vi "Temp PID Control.vi"() -> ()   [LabVIEW 2018]
doc: "This example demonstrates how to generate digital output data using software timing.\n\nFor instructions on how to connect your signals from the DAQ device, refer to your device documentation."
uses:
  <vilib>/Utility/error.llb/DialogType.ctl
  <vilib>/DAQmx/write.llb/DAQmx Write (Digital Bool 1Line 1Point).vi
  <vilib>/DAQmx/create/channels.llb/DAQmx Create Channel (AI-Voltage-Basic).vi
  <vilib>/DAQmx/configure/timing.llb/DAQmx Timing (Sample Clock).vi
  <resource>/objmgr/daqmx.rc
  <vilib>/DAQmx/read.llb/DAQmx Read (Analog Wfm 1Chan NSamp).vi
  <vilib>/measure/NI_MAPro.lvlib
  <vilib>/measure/madcrms.llb/Basic Averaged DC-RMS for 1 Chan.vi
  <vilib>/addons/control/pid/NI_PID_pid.lvlib
  <vilib>/addons/control/pid/pid.llb/PID (DBL).vi
  <vilib>/DAQmx/create/channels.llb/DAQmx Create Channel (DO-Digital Output).vi
  <vilib>/DAQmx/write.llb/DAQmx Write (Digital 1D Bool NChan 1Samp 1Line).vi
panel:
  out "STOP":bool
  out "On Ratio [%]":dbl format="%.2f"
  in  "output range":cluster{"output high":dbl, "output low":dbl}={"output high"=100.0, "output low"=0.0} {"output low" format="%.2f"; "output high" format="%.2f"}
  in  "PID gains":T1={"proportional gain (Kc)"=1.0, "integral time (Ti, min)"=0.01, "derivative time (Td, min)"=0.0} {"derivative time (Td, min)" format="%.3f"; "integral time (Ti, min)" format="%.3f"; "proportional gain (Kc)" format="%.3f"}
  in  "Temperature Setpoint":dbl(slide) scale=20.0..100.0
  out "Average Temperature":dbl=1000.0 format="%0.2f"
  in  "Temperature Window Length in [s]":dbl=1000.0
  out "Waveform Graph":waveform(dbl)(graph)
  in  "Sample Rate":dbl=1000.0
  in  "Sample Clock Source":tag="OnboardClock"
  in  "Terminal Configuration":i32(ring)=-1 items=["default"=-1, "RSE"=10083, "NRSE"=10078, "Differential"=10106, "Pseudodifferential"=12529]
  in  "Max Voltage":dbl=5.0
  in  "Min Voltage":dbl=-5.0
  in  "Physical Channel":tag="Dev1/ai0"
  out "Actual Sample Rate":dbl=1000.0 format="%0.2f"
  in  "Stop":bool
  in  "Line(s)":tag="Dev1/port0/line0:1"
  # "Digital Output Channel"
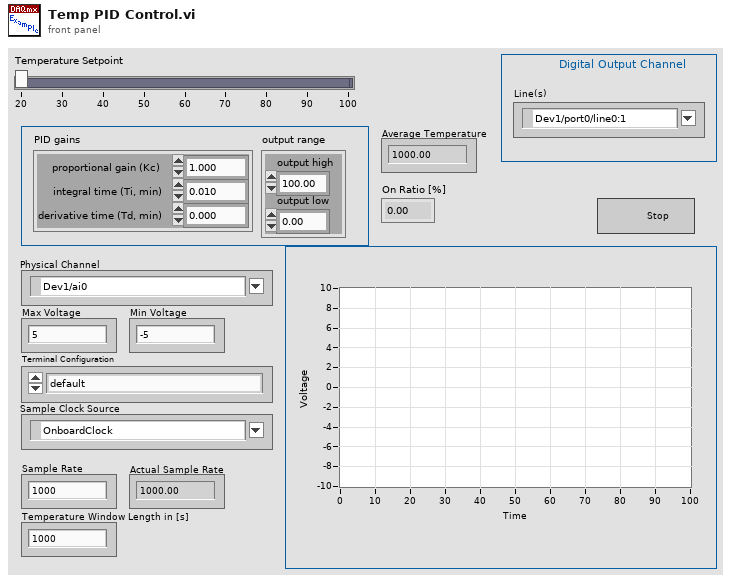
[diagram p1: front panel]
types:
  T1 = cluster{"proportional gain (Kc)":dbl, "integral time (Ti, min)":dbl, "derivative time (Td, min)":dbl}
  T2 = typedef "DialogType.ctl" = u16
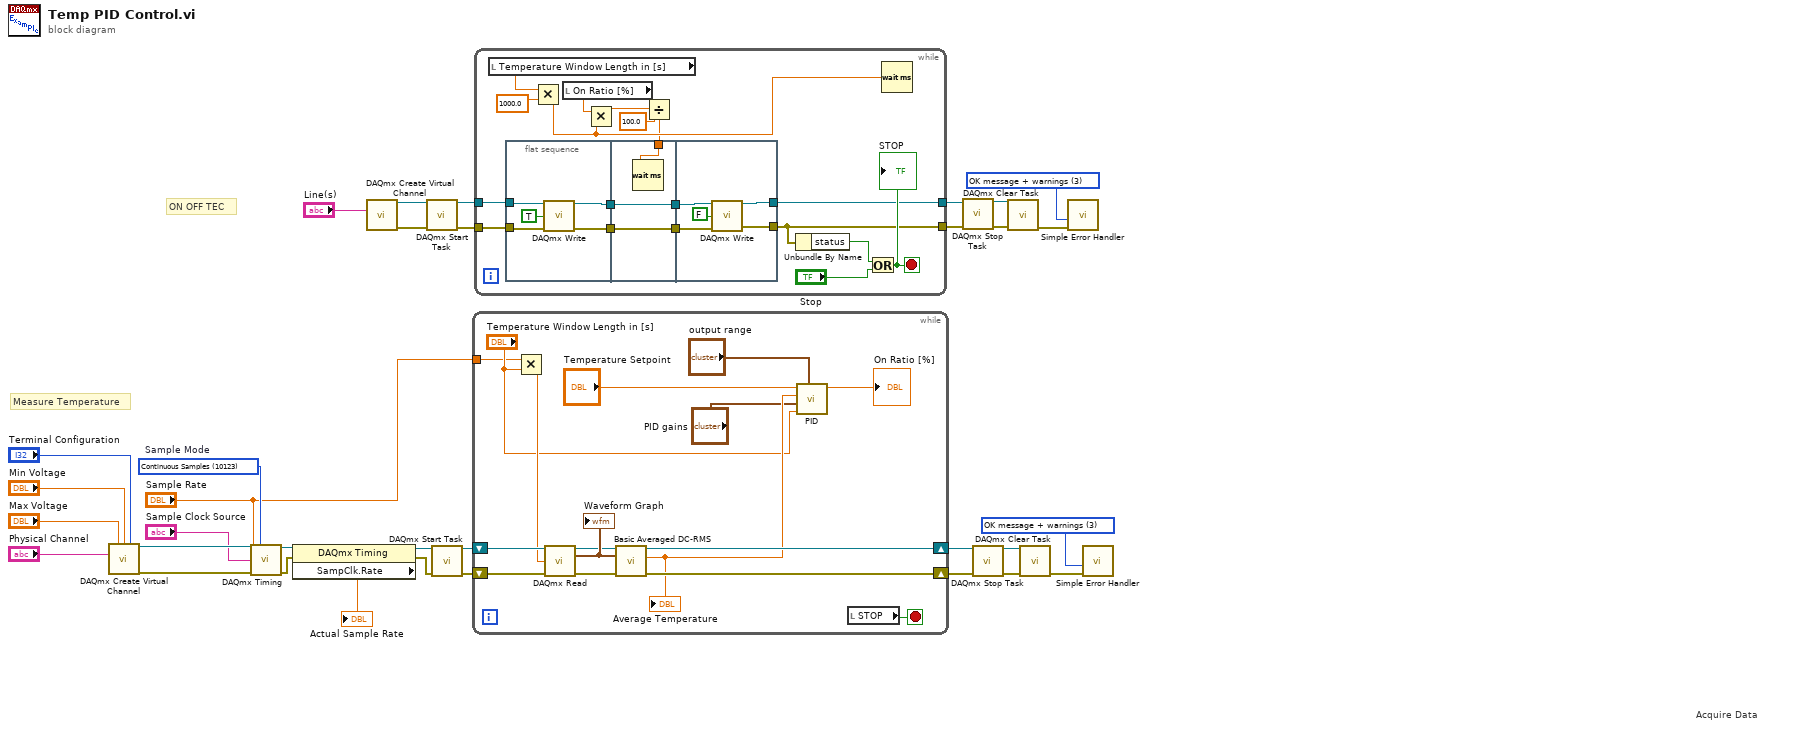
[diagram p0: block diagram]
diagram:
  w4 = T2 3 items=["no dialog", "OK message", "continue or stop message", "OK message + warnings", "continue/stop + warnings"] ("type of dialog (OK msg:1)")
  w20 = 10123 items=["Finite Samples"=10178, "Continuous Samples"=10123, "Hardware Timed Single Point"=12522]  # Sample Mode
  w25 = T2 3 items=["no dialog", "OK message", "continue or stop message", "OK message + warnings", "continue/stop + warnings"] ("type of dialog (OK msg:1)")
  # "Measure Temperature"
  # "ON OFF TEC"
  # "Acquire Data"
  n1 = call-poly <vilib>:"DAQmx Create Virtual Channel.vi"("maximum value"="Max Voltage", "minimum value"="Min Voltage", "input terminal configuration"="Terminal Configuration", "physical channels"="Physical Channel") -> ("task out"=w18:refnum<k21>, "error out"=w19:errorcluster)  [unwired: 10 in]
  n2 = call-poly <vilib>:"DAQmx Timing.vi"("task/channels in"=w18, "sample mode"=w20, "rate"="Sample Rate", "source"="Sample Clock Source", "error in"=w19) -> ("task out"=w22:refnum<k21>, "error out"=w21:errorcluster)  [unwired: 9 in]
  n3 = property class="DAQmx Timing"(reference=w22, error in=w21) -> (reference out=w3:refnum<k21>, error out=w2:errorcluster, "SampClk.Rate"=→"Actual Sample Rate":dbl)
  n4 = call-poly <vilib>:"DAQmx Create Virtual Channel.vi"("lines"="Line(s)") -> ("task out"=w28:refnum<k21>, "error out"=w29:errorcluster)  [unwired: 13 in]
  n5 = call <vilib>:"DAQmx Start Task.vi"("task/channels in"=w28, "error in"=w29) -> ("task out"=w33:refnum<k21>, "error out"=w32:errorcluster)  [unwired: 12 in]
  n6 = call <vilib>:"DAQmx Start Task.vi"("task/channels in"=w3, "error in"=w2) -> ("task out"=w17:refnum<k21>, "error out"=w16:errorcluster)  [unwired: 12 in]
  n7 = while {
    shift-right: [w42] -> w6
    shift-left: w17 -> [w48]
    shift-right: [w43] -> w5
    shift-left: w16 -> [w47]
    tunnel: "Sample Rate" -> [w35]
    stop <- w34 stop-if-true
    n8 = Multiply(x=w35, y="Temperature Window Length in [s]") -> (x*y=w46:dbl)
    n9 = call-poly <vilib>:"DAQmx Read.vi"("task/channels in"=w48, "number of samples per channel"=w46, "error in"=w47) -> ("task out"=w42:refnum<k21>, "data"=w44:waveform(dbl), "error out"=w45:errorcluster)  [unwired: 10 in]
    "Waveform Graph" <- w44
    n10 = call-poly <vilib>:"Basic Averaged DC-RMS.vi"("error in (no error)"=w45, "signal in"=w44) -> ("error out"=w43:errorcluster, "DC value"=w40:dbl)  [unwired: 6 in, 2 out]
    "Average Temperature" <- w40
    n11 = call-poly <vilib>:"PID.vi"("output range"="output range", "dt (s)"="Temperature Window Length in [s]", "PID gains"="PID gains", "process variable"=w40, "setpoint"="Temperature Setpoint") -> ("output"=→"On Ratio [%]":dbl)  [unwired: 5 in, 1 out]
    n12 = local read "STOP"() -> (w34:bool)
  }
  n13 = while {
    tunnel: w33 -> [w66]
    tunnel: w32 -> [w65]
    tunnel: [w57] -> w24
    tunnel: [w56] -> w23
    stop <- w64 stop-if-true
    n14 = local read "Temperature Window Length in [s]"() -> (w49:dbl)
    n15 = flat-sequence {
      tunnel: w66 -> [w70]
      tunnel: w65 -> [w69]
      tunnel: [w68] -> w60
      tunnel: [w67] -> w58
      tunnel: [w74] -> w61
      tunnel: w60 -> [w74]
      tunnel: [w73] -> w59
      tunnel: w58 -> [w73]
      tunnel: w51 -> [w72]
      tunnel: w61 -> [w79]
      tunnel: w59 -> [w78]
      tunnel: [w77] -> w57
      tunnel: [w76] -> w56
      frame #0 {
        n16 = call-poly <vilib>:"DAQmx Write.vi"("task/channels in"=w70, "data"=TRUE, "error in"=w69) -> ("task out"=w68:refnum<k21>, "error out"=w67:errorcluster)  [unwired: 10 in, 1 out]
      }
      frame #1 {
        n17 = Wait (ms)(milliseconds to wait=w72) -> ()  [unwired: 1 out]
      }
      frame #2 {
        n18 = call-poly <vilib>:"DAQmx Write.vi"("task/channels in"=w79, "data"=FALSE, "error in"=w78) -> ("task out"=w77:refnum<k21>, "error out"=w76:errorcluster)  [unwired: 10 in, 1 out]
      }
    }
    n19 = Multiply(x=w49, y=1000.0) -> (x*y=w54:dbl)
    n20 = local read "On Ratio [%]"() -> (w50:dbl)
    n21 = Multiply(x=w50, y=w54) -> (x*y=w53:dbl)
    n22 = Divide(x=w53, y=100.0) -> (x/y=w51:dbl)
    n23 = Unbundle By Name(w56) -> ("status"=w63:bool)
    n24 = Or(x=w63, y="Stop") -> (x .or. y?=w64:bool)
    "STOP" <- w64
    n25 = Wait (ms)(milliseconds to wait=w54) -> ()  [unwired: 1 out]
  }
  n26 = call <vilib>:"DAQmx Stop Task.vi"("task/channels in"=w24, "error in"=w23) -> ("task out"=w27:refnum<k21>, "error out"=w26:errorcluster)  [unwired: 12 in]
  n27 = call <vilib>:"DAQmx Stop Task.vi"("task/channels in"=w6, "error in"=w5) -> ("task out"=w8:refnum<k21>, "error out"=w7:errorcluster)  [unwired: 12 in]
  n28 = call <vilib>:"DAQmx Clear Task.vi"("task in"=w27, "error in"=w26) -> ("error out"=w31:errorcluster)  [unwired: 13 in]
  n29 = call <vilib>:"DAQmx Clear Task.vi"("task in"=w8, "error in"=w7) -> ("error out"=w15:errorcluster)  [unwired: 13 in]
  n30 = call <vilib>:"Simple Error Handler.vi"("type of dialog (OK msg:1)"=w25, "error in (no error)"=w31) -> ()  [unwired: 3 in, 5 out]
  n31 = call <vilib>:"Simple Error Handler.vi"("type of dialog (OK msg:1)"=w4, "error in (no error)"=w15) -> ()  [unwired: 3 in, 5 out]
